vi "CALIBRATION_SUMMARY.vi"(0 "flow_slope_IN":dbl=50.0 format="%.2f", 1 "flow_slope_OUT":dbl=56.0 format="%.2f", 2 "Path":path=path "C:/KPRO_2010/Output_files/slopes-cal-record.txt", 3 "pressure_slope_OUT":dbl=23.33 format="%.2f", 5 "pressure_slope_IN":dbl=23.33 format="%.2f", 9 "string_pot_slope_IN":dbl=1.5 format="%.2f", 11 "error in (no error)":errorcluster, 12 "string_pot_slope_OUT":dbl=1.5 format="%.2f") -> (15 "error out":errorcluster)   [LabVIEW 2016]
uses:
  <userlib>/_OpenG.lib/file/file.llb/Strip Path - Traditional__ogtk.vi
  <userlib>/_OpenG.lib/file/file.llb/Build Path - Traditional__ogtk.vi
  <vilib>/Utility/file.llb/Write Delimited Spreadsheet (string).vi
  Kpro Globals.vi
  <vilib>/Utility/file.llb/Write Delimited Spreadsheet (DBL).vi
panel:
  out "test slopes file":path
  out "Record Output Slopes to File":path
  out "KPRO Box Number":dbl=800.0
  out "Date_and_time":string
  out "pressure_slope_OUT 2":dbl=23.33 format="%.2f"
  out "flow_slope_OUT 2":dbl=51.35 format="%.2f"
  out "string_pot_slope_OUT 2":dbl=1.5 format="%.2f"
  out "pressure_slope_IN 2":dbl=23.33 format="%.2f"
  out "flow_slope_IN 2":dbl=51.35 format="%.2f"
  out "string_pot_slope_IN 2":dbl=1.5 format="%.2f"
  in  "ok":bool
  # "CALIBRATION SUMMARY"
  # "Record these values in Kpro Box Calibration Log"
  # "DATE"
  # "TIME"
  # "Initial Slope              New Slope"
  # "Flow Sensor"
  # "mL/min/V"
  # "Up hole\nPressure Transducer"
  # "ft/V"
  # "String Potentiometer"
  # "ft/V"
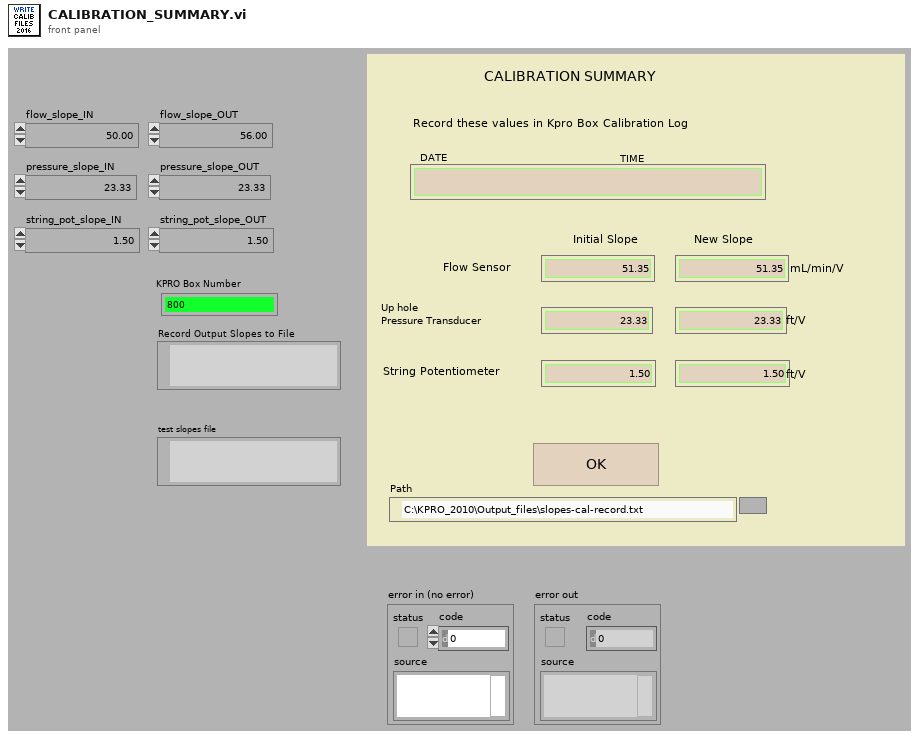
[diagram p1: front panel]
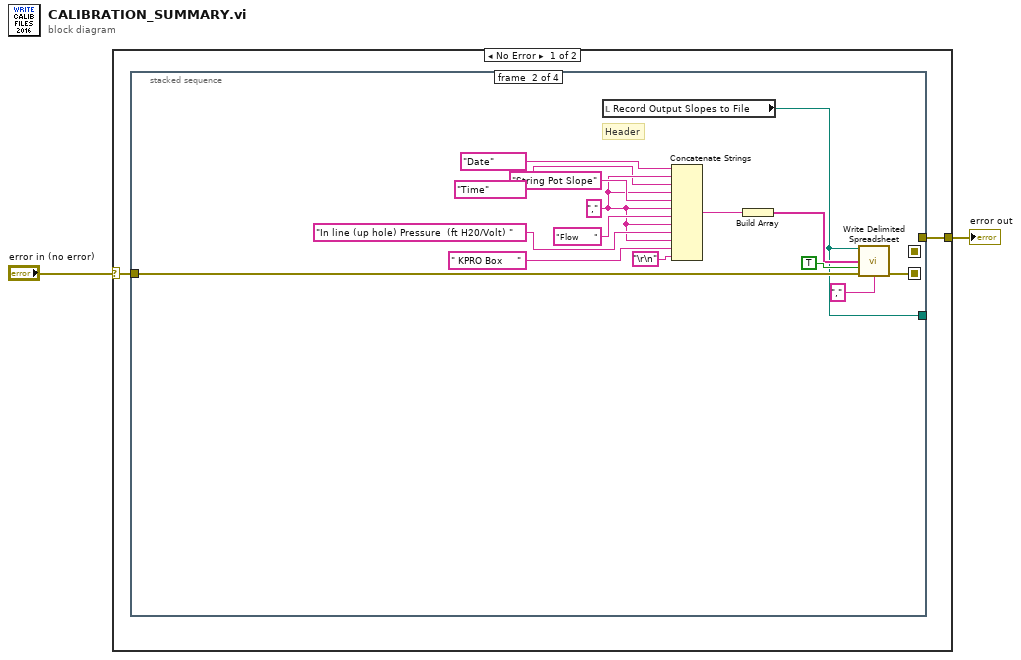
[diagram p0: block diagram]
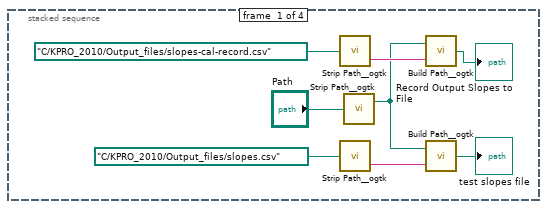
[diagram p2: hidden frame]
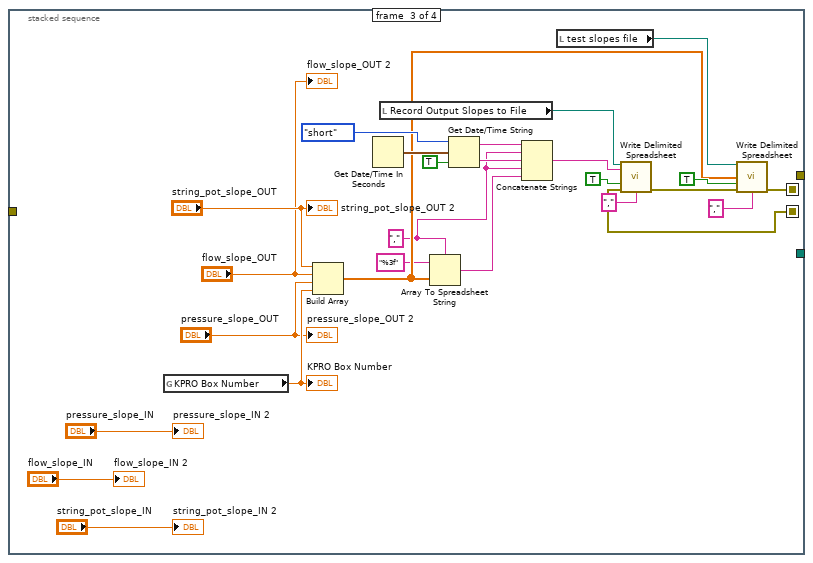
[diagram p3: hidden frame]
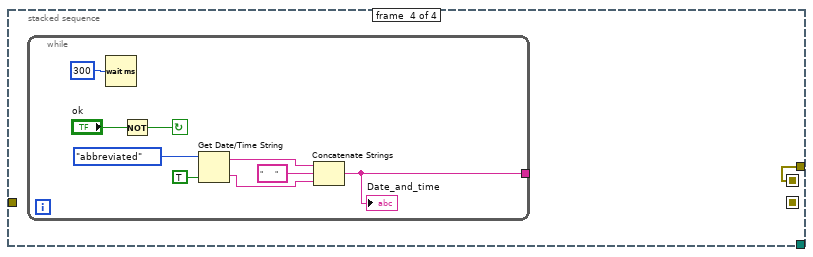
[diagram p4: hidden frame]
diagram:
  n1 = case shown="No Error" "error in (no error)" {
    selector: "error in (no error)" -> [w4 w64]
    tunnel: [w3 w64] -> w2
    frame No Error {
      n2 = stacked-sequence {
        seq-local: [_ w18 _ _] -> [_ _ w34 _]
        seq-local: [_ _ w45 _] -> [_ _ _ w54]
        tunnel: w4 -> [_ w21 _ _]
        tunnel: [_ _ _ w54] -> w3
        tunnel: [_ w13 _ _] -> _
        frame #0 {
          n3 = call-poly <userlib>:"Strip Path__ogtk.vi"("path"=path "C:/KPRO_2010/Output_files/slopes-cal-record.csv") -> ("name"=w11:string)  [unwired: 1 out]
          n4 = call-poly <userlib>:"Strip Path__ogtk.vi"("path"=path "C:/KPRO_2010/Output_files/slopes.csv") -> ("name"=w8:string)  [unwired: 1 out]
          n5 = call-poly <userlib>:"Strip Path__ogtk.vi"("path"="Path") -> ("stripped path"=w9:path)  [unwired: 1 out]
          n6 = call-poly <userlib>:"Build Path__ogtk.vi"("name or relative path"=w11, "base path"=w9) -> ("appended path"=→"Record Output Slopes to File":path)
          n7 = call-poly <userlib>:"Build Path__ogtk.vi"("name or relative path"=w8, "base path"=w9) -> ("appended path"=→"test slopes file":path)
        }
        frame #1 {
          w16 = "," ("string")
          # "Header"
          n8 = local read "Record Output Slopes to File"() -> (w13:path)
          n9 = Concatenate Strings("Date" ("string"), w16, "Time" ("string"), w16, "String Pot Slope" ("string"), w16, "Flow     " ("string"), w16, "In line (up hole) Pressure  (ft H20/Volt) " ("string"), w16, " KPRO Box     " ("string"), "\r\n") -> (w20:string)
          n10 = Build Array(w20) -> (w19:string[])
          n11 = call-poly <vilib>:"Write Delimited Spreadsheet.vi"("file path (dialog if empty)"=w13, "1D data"=w19, "append to file? (new file:F)"=TRUE, "error in (no error)"=w21, "delimiter (\\t)"="," ("delimiter (\\t)")) -> ("error out"=w18:errorcluster)  [unwired: 9 in, 1 out]
        }
        frame #2 {
          w29 = "," ("delimiter (\\t)")
          n12 = global read "Kpro Globals.vi" "KPRO Box Number"() -> (w48:dbl)
          "KPRO Box Number" <- w48
          n13 = Build Array("string_pot_slope_OUT", "flow_slope_OUT", "pressure_slope_OUT", w48) -> (w39:dbl[])
          n14 = Get Date/Time In Seconds() -> (seconds since 1Jan1904=w41:timestamp)
          n15 = local read "Record Output Slopes to File"() -> (w37:path)
          n16 = Array To Spreadsheet String(delimiter (Tab)=w29, array=w39, 3:"%3f" ("format string")) -> (spreadsheet string=w30:string)
          n17 = Get Date/Time String(date format (0)=enum16{"short", "long", "abbreviated"}."short", seconds (now)=w41, want seconds? (F)=TRUE) -> (date string=w31:string, time string=w32:string)
          n18 = Concatenate Strings(w31, w29, w32, w29, w30) -> (w33:string)
          n19 = local read "test slopes file"() -> (w44:path)
          n20 = call-poly <vilib>:"Write Delimited Spreadsheet.vi"("file path (dialog if empty)"=w37, "format (%.3f)"=w33, "append to file? (new file:F)"=TRUE, "error in (no error)"=w34, "delimiter (\\t)"="," ("delimiter (\\t)")) -> ("error out"=w35:errorcluster)  [unwired: 9 in, 1 out]
          n21 = call-poly <vilib>:"Write Delimited Spreadsheet.vi"("file path (dialog if empty)"=w44, "1D data"=w39, "append to file? (new file:F)"=TRUE, "error in (no error)"=w35, "delimiter (\\t)"="," ("delimiter (\\t)")) -> ("error out"=w45:errorcluster)  [unwired: 9 in, 1 out]
          "pressure_slope_IN 2" <- "pressure_slope_IN"
          "flow_slope_IN 2" <- "flow_slope_IN"
          "string_pot_slope_IN 2" <- "string_pot_slope_IN"
          "pressure_slope_OUT 2" <- "pressure_slope_OUT"
          "flow_slope_OUT 2" <- "flow_slope_OUT"
          "string_pot_slope_OUT 2" <- "string_pot_slope_OUT"
        }
        frame #3 {
          n22 = while {
            tunnel: [w55] -> _
            stop <- w63 continue-if-true
            n23 = Wait (ms)(milliseconds to wait=u32 300) -> ()  [unwired: 1 out]
            n24 = Not(x="ok") -> (.not. x?=w63:bool)
            n25 = Get Date/Time String(date format (0)=enum16{"short", "long", "abbreviated"}."abbreviated", want seconds? (F)=TRUE) -> (date string=w60:string, time string=w57:string)  [unwired: 1 in]
            n26 = Concatenate Strings(w60, "      " ("string"), w57) -> (w55:string)
            "Date_and_time" <- w55
          }
        }
      }
    }
    frame Error {
    }
  }
  "error out" <- w2
